vi "CRYNameChecking.vi"(0 "Curve Name":string, 2 "Mode":i8, 3 "Work in":u16) -> (9 "Out Calcurated":bool)   [LabVIEW 2013]
uses:
  CRYStatistics Global.vi
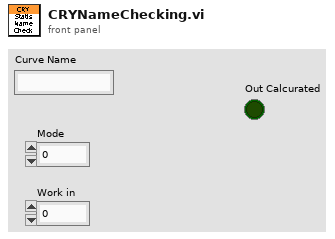
[diagram p1: front panel]
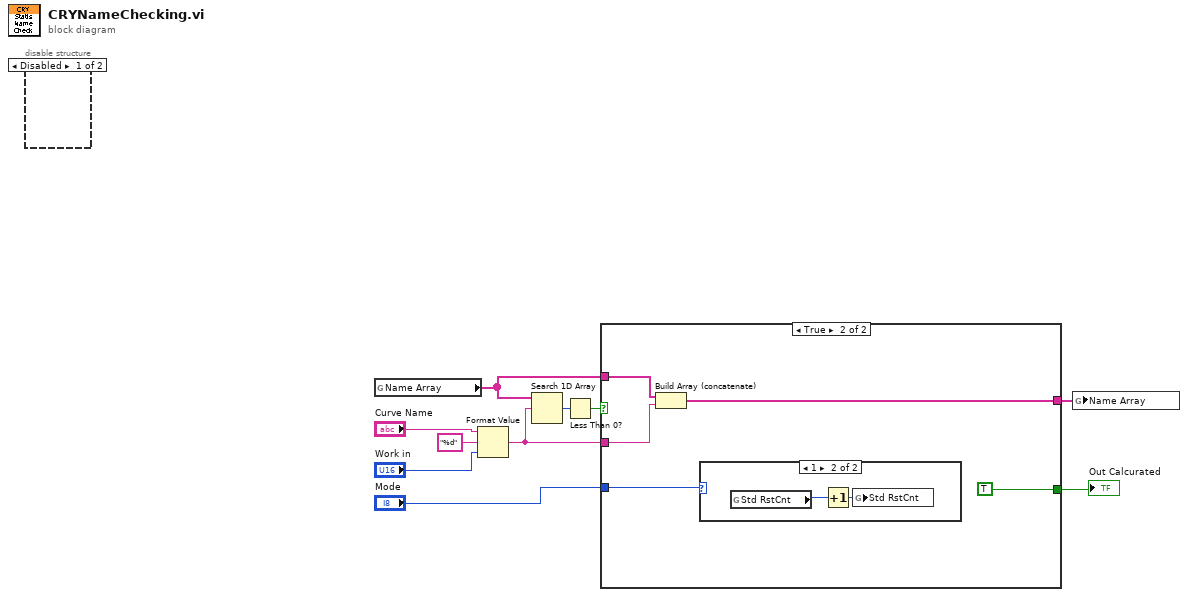
[diagram p0: block diagram]
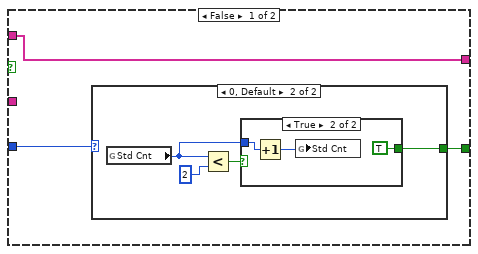
[diagram p2: hidden frame]
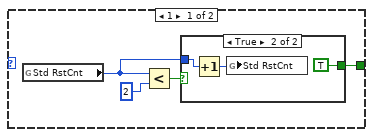
[diagram p3: hidden frame]
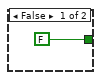
[diagram p4: hidden frame]
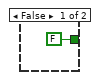
[diagram p5: hidden frame]
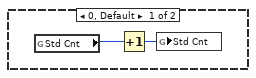
[diagram p6: hidden frame]
diagram:
  n1 = disable-structure shown="Disabled" {
    frame Disabled {
    }
    frame Enabled {
    }
  }
  n2 = global read "CRYStatistics Global.vi" "Name Array"() -> (w7:string[])
  n3 = Format Value(string ("")="Curve Name", format string="%d", value (0)="Work in") -> (output string=w1:string)
  n4 = Search 1D Array(1D array=w7, element=w1) -> (index of element=w9:i32)  [unwired: 1 in]
  n5 = Less Than 0?(x=w9) -> (x < 0?=w8:bool)
  n6 = case shown="True" w8 {
    tunnel: w7 -> [w13 w34]
    tunnel: [w13 w33] -> w6
    tunnel: [w12 TRUE] -> w10
    tunnel: "Mode" -> [w11 w31]
    tunnel: w1 -> [_ w30]
    frame False {
      n7 = case shown="0, Default" w11 {
        tunnel: [w14 w22] -> w12
        frame 1 {
          n8 = global read "CRYStatistics Global.vi" "Std RstCnt"() -> (w15:u32)
          n9 = Less?(x=w15, y=u32 2) -> (x < y?=w16:bool)
          n10 = case shown="True" w16 {
            tunnel: w15 -> [_ w20]
            tunnel: [FALSE TRUE] -> w14
            frame False {
            }
            frame True {
              n11 = Increment(x=w20) -> (x+1=w21:u32)
              n12 = global write "CRYStatistics Global.vi" "Std RstCnt"(w21) -> ()
            }
          }
        }
        frame 0, Default {
          n13 = global read "CRYStatistics Global.vi" "Std Cnt"() -> (w23:u32)
          n14 = Less?(x=w23, y=u32 2) -> (x < y?=w24:bool)
          n15 = case shown="True" w24 {
            tunnel: w23 -> [_ w28]
            tunnel: [FALSE TRUE] -> w22
            frame False {
            }
            frame True {
              n16 = Increment(x=w28) -> (x+1=w29:u32)
              n17 = global write "CRYStatistics Global.vi" "Std Cnt"(w29) -> ()
            }
          }
        }
      }
    }
    frame True {
      n18 = Build Array (concatenate)(w34, w30) -> (w33:string[])
      n19 = case shown="1" w31 {
        frame 0, Default {
          n20 = global read "CRYStatistics Global.vi" "Std Cnt"() -> (w36:u32)
          n21 = Increment(x=w36) -> (x+1=w35:u32)
          n22 = global write "CRYStatistics Global.vi" "Std Cnt"(w35) -> ()
        }
        frame 1 {
          n23 = global read "CRYStatistics Global.vi" "Std RstCnt"() -> (w38:u32)
          n24 = Increment(x=w38) -> (x+1=w37:u32)
          n25 = global write "CRYStatistics Global.vi" "Std RstCnt"(w37) -> ()
        }
      }
    }
  }
  "Out Calcurated" <- w10
  n26 = global write "CRYStatistics Global.vi" "Name Array"(w6) -> ()
